vi "JPL Solenoid Block.vi"(8 "Boolean Inputs":T2, 11 "References":T3) -> (2 "Status Outputs":T1)   [LabVIEW 2015]
uses:
  <vilib>/functionblocks/Counter/Pulse Timer/Pulse Timer.vi
  <vilib>/Rock Robotics/WPI/Solenoid/Deprecated/WPI_SolenoidSetBool.vi
  <vilib>/functionblocks/FB Core/FB Core.xnode
  <vilib>/functionblocks/NI_FunctionBlock Libraries.lvlib
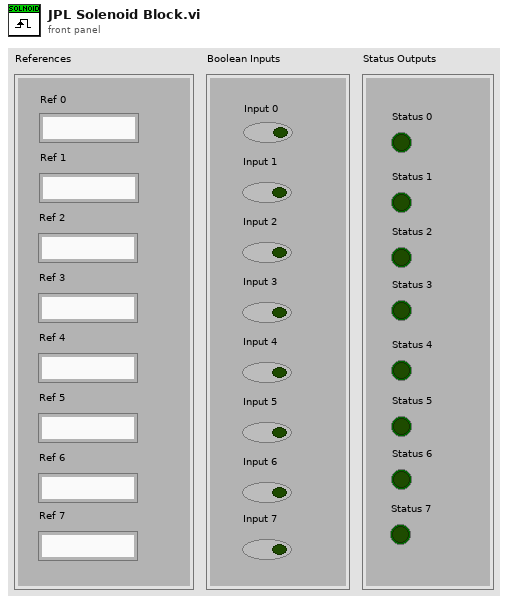
[diagram p1: front panel]
types:
  T1 = cluster{"Status 0":bool, "Status 1":bool, "Status 2":bool, "Status 3":bool, "Status 4":bool, "Status 5":bool, "Status 6":bool, "Status 7":bool}
  T2 = cluster{"Input 0":bool, "Input 1":bool, "Input 2":bool, "Input 3":bool, "Input 4":bool, "Input 5":bool, "Input 6":bool, "Input 7":bool}
  T3 = cluster{"Ref 7":string, "Ref 6":string, "Ref 5":string, "Ref 4":string, "Ref 3":string, "Ref 2":string, "Ref 1":string, "Ref 0":string}
  T4 = typedef "WPI_SolenoidDevRef.ctl" = cluster{"DevStatus":errorcluster, "Pneumatics Control Module":u8, "Forward Solenoid Channel":T5, "Reverse Solenoid Channel":T5}
  T5 = typedef "WPI_SolenoidChannel.ctl" = enum8{"Solenoid 0", "Solenoid 1", "Solenoid 2", "Solenoid 3", "Solenoid 4", "Solenoid 5", "Solenoid 6", "Solenoid 7", "Invalid"}
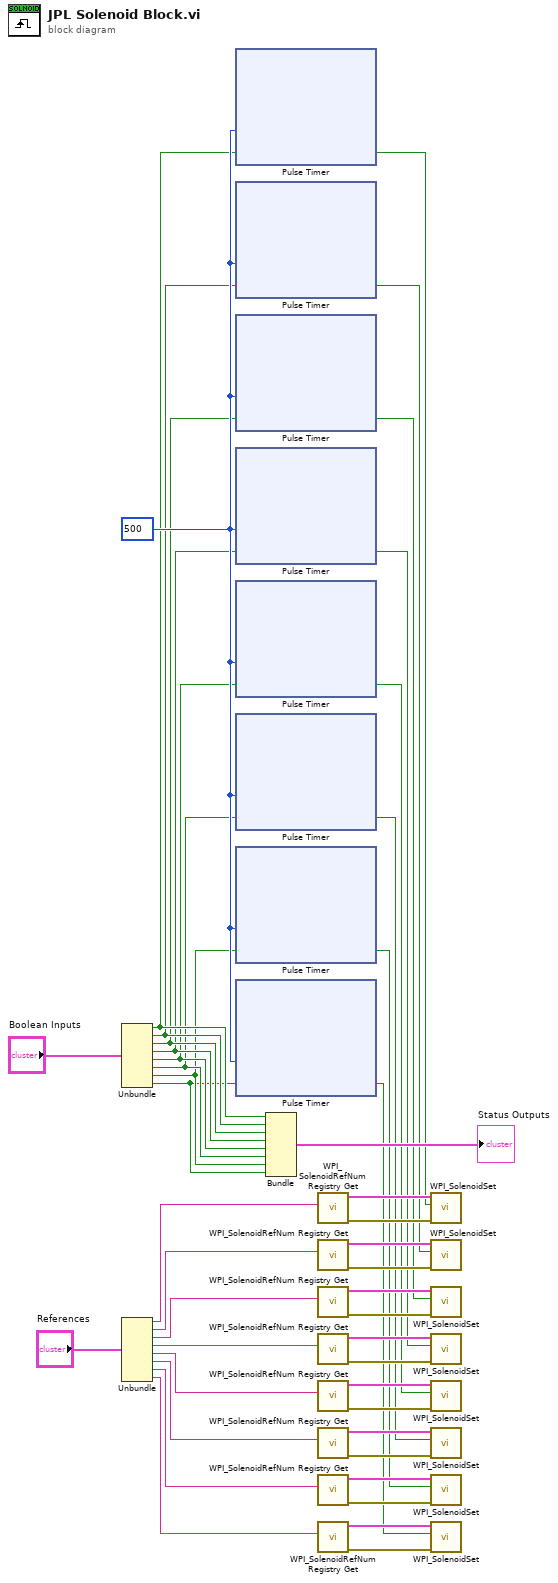
[diagram p0: block diagram]
diagram:
  w9 = 500
  n1 = Unbundle("Boolean Inputs") -> ("Input 0"=w8:bool, "Input 1"=w7:bool, "Input 2"=w6:bool, "Input 3"=w5:bool, "Input 4"=w4:bool, "Input 5"=w3:bool, "Input 6"=w2:bool, "Input 7"=w1:bool)
  n2 = Unbundle("References") -> ("Ref 7"=w25:string, "Ref 6"=w24:string, "Ref 5"=w23:string, "Ref 4"=w22:string, "Ref 3"=w21:string, "Ref 2"=w20:string, "Ref 1"=w19:string, "Ref 0"=w18:string)
  n3 = xnode "Pulse Timer"("preset time (ms)"=w9, "input"=w8) -> ("output"=w17:bool)  [unwired: 1 in, 2 out]
  n4 = xnode "Pulse Timer"("preset time (ms)"=w9, "input"=w7) -> ("output"=w16:bool)  [unwired: 1 in, 2 out]
  n5 = xnode "Pulse Timer"("preset time (ms)"=w9, "input"=w6) -> ("output"=w15:bool)  [unwired: 1 in, 2 out]
  n6 = xnode "Pulse Timer"("preset time (ms)"=w9, "input"=w5) -> ("output"=w14:bool)  [unwired: 1 in, 2 out]
  n7 = xnode "Pulse Timer"("preset time (ms)"=w9, "input"=w4) -> ("output"=w13:bool)  [unwired: 1 in, 2 out]
  n8 = xnode "Pulse Timer"("preset time (ms)"=w9, "input"=w3) -> ("output"=w12:bool)  [unwired: 1 in, 2 out]
  n9 = xnode "Pulse Timer"("preset time (ms)"=w9, "input"=w2) -> ("output"=w11:bool)  [unwired: 1 in, 2 out]
  n10 = xnode "Pulse Timer"("preset time (ms)"=w9, "input"=w1) -> ("output"=w10:bool)  [unwired: 1 in, 2 out]
  n11 = Bundle("Input 0"=w8, "Input 1"=w7, "Input 2"=w6, "Input 3"=w5, "Input 4"=w4, "Input 5"=w3, "Input 6"=w2, "Input 7"=w1) -> (→"Status Outputs":T2)  [unwired: 1 in]
  n12 = call <vilib>:"WPI_SolenoidRefNum Registry Get.vi"("refnum name"=w25) -> ("error out"=w43:errorcluster, "SolenoidDevRef"=w44:T4)  [unwired: 9 in]
  n13 = call <vilib>:"WPI_SolenoidRefNum Registry Get.vi"("refnum name"=w24) -> ("error out"=w41:errorcluster, "SolenoidDevRef"=w42:T4)  [unwired: 9 in]
  n14 = call <vilib>:"WPI_SolenoidRefNum Registry Get.vi"("refnum name"=w23) -> ("error out"=w39:errorcluster, "SolenoidDevRef"=w40:T4)  [unwired: 9 in]
  n15 = call <vilib>:"WPI_SolenoidRefNum Registry Get.vi"("refnum name"=w22) -> ("error out"=w34:errorcluster, "SolenoidDevRef"=w35:T4)  [unwired: 9 in]
  n16 = call <vilib>:"WPI_SolenoidRefNum Registry Get.vi"("refnum name"=w21) -> ("error out"=w32:errorcluster, "SolenoidDevRef"=w33:T4)  [unwired: 9 in]
  n17 = call <vilib>:"WPI_SolenoidRefNum Registry Get.vi"("refnum name"=w20) -> ("error out"=w30:errorcluster, "SolenoidDevRef"=w31:T4)  [unwired: 9 in]
  n18 = call <vilib>:"WPI_SolenoidRefNum Registry Get.vi"("refnum name"=w19) -> ("error out"=w28:errorcluster, "SolenoidDevRef"=w29:T4)  [unwired: 9 in]
  n19 = call <vilib>:"WPI_SolenoidRefNum Registry Get.vi"("refnum name"=w18) -> ("error out"=w26:errorcluster, "SolenoidDevRef"=w27:T4)  [unwired: 9 in]
  n20 = call-poly <vilib>:"WPI_SolenoidSet.vi"("error in (no error)"=w43, "Value"=w17, "SolenoidDevRef"=w44) -> ()  [unwired: 7 in, 2 out]
  n21 = call-poly <vilib>:"WPI_SolenoidSet.vi"("error in (no error)"=w41, "Value"=w16, "SolenoidDevRef"=w42) -> ()  [unwired: 7 in, 2 out]
  n22 = call-poly <vilib>:"WPI_SolenoidSet.vi"("error in (no error)"=w39, "Value"=w15, "SolenoidDevRef"=w40) -> ()  [unwired: 7 in, 2 out]
  n23 = call-poly <vilib>:"WPI_SolenoidSet.vi"("error in (no error)"=w34, "Value"=w14, "SolenoidDevRef"=w35) -> ()  [unwired: 7 in, 2 out]
  n24 = call-poly <vilib>:"WPI_SolenoidSet.vi"("error in (no error)"=w32, "Value"=w13, "SolenoidDevRef"=w33) -> ()  [unwired: 7 in, 2 out]
  n25 = call-poly <vilib>:"WPI_SolenoidSet.vi"("error in (no error)"=w30, "Value"=w12, "SolenoidDevRef"=w31) -> ()  [unwired: 7 in, 2 out]
  n26 = call-poly <vilib>:"WPI_SolenoidSet.vi"("error in (no error)"=w28, "Value"=w11, "SolenoidDevRef"=w29) -> ()  [unwired: 7 in, 2 out]
  n27 = call-poly <vilib>:"WPI_SolenoidSet.vi"("error in (no error)"=w26, "Value"=w10, "SolenoidDevRef"=w27) -> ()  [unwired: 7 in, 2 out]
